vi "Load-lasing-files.vi"(8 "error in (no error)":errorcluster, 11 "Object ref in":T1) -> (0 "error out":errorcluster, 3 "Object ref out":T1)   [LabVIEW 2013, in "SLMControl.lvlib" / "SC-Main.lvclass"]
uses:
  SC-Main.lvclass
  Object-reference.ctl
  SC-Main.lvclass/SC-Main.ctl
  Application-status.ctl
  UI/Control-names.ctl
  Read UI.vi
  Read Status.vi
  Read Base path.vi
  UI/Set-control-boolean.vi
  UI/Set-control-enable-single.vi
  UI/SC-UI.lvclass
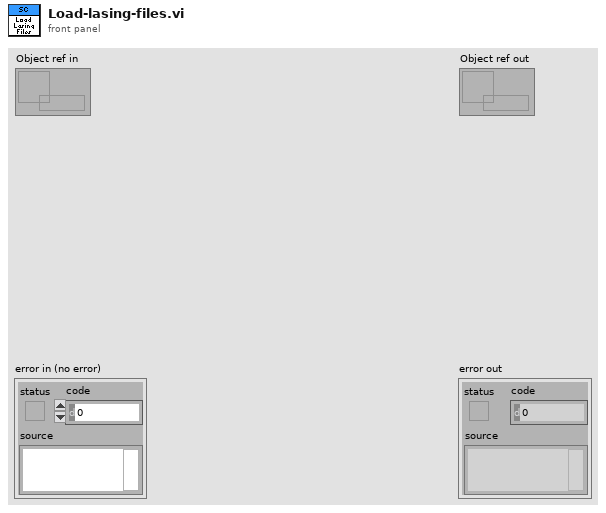
[diagram p1: front panel]
types:
  T1 = typedef "SLMControl.lvlib/SC-Main.lvclass/Object-reference.ctl" = refnum<data-value>
  T2 = typedef "SLMControl.lvlib/SC-UI.lvclass/Control-names.ctl" = enum16{"Com-in", "Com-out", "Help", "Status", "Load configuration", "Save configuration", "Load lasing files", "Load deposition files", "Clear", "Files", "Activate", "Execute", "Abort", "Options", "Current layer", "Current iteration", "Last elapsed time", "Deposition status", "Lasing job", "Status LEDs", "Exiting led", "Initialized led", "Files loaded led", "Activated led", "Executing led", "Deposition led", "Lasing job led", "Lasing led"}
  T3 = typedef "SLMControl.lvlib/SC-Main.lvclass/Application-status.ctl" = enum16{"Idle", "Initialized", "Configured", "Activated", "Started", "Paused", "Stopped", "Reset", "Error", "Exited"}
  T4 = typedef "SLMControl.lvlib/SC-UI.lvclass/Panes-reference.ctl" = refnum<data-value>
  T5 = typedef "SLMControl.lvlib/SC-Main.lvclass/Client-status.ctl" = enum16{"Idle", "Initialized", "Configured", "Activated", "Started", "Paused", "Stopped", "Reset", "Error", "Exited"}
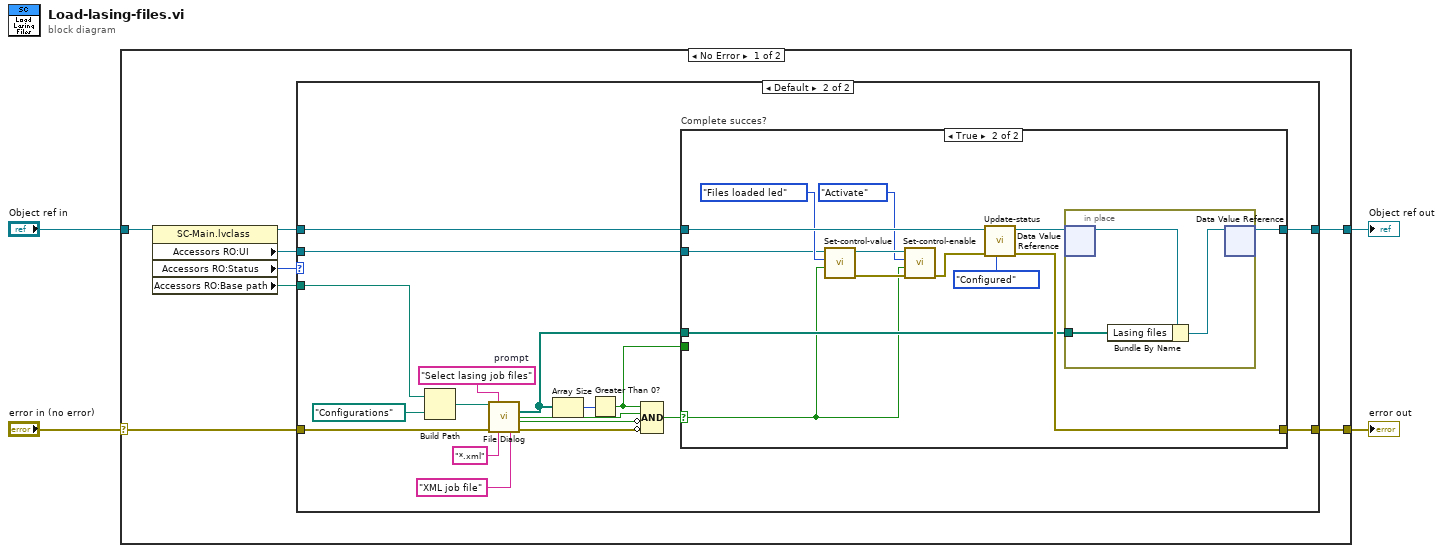
[diagram p0: block diagram]
diagram:
  n1 = case shown="No Error" "error in (no error)" {
    selector: "error in (no error)" -> [w12 w51]
    tunnel: [w8 w51] -> w3
    tunnel: [w7 w50] -> w1
    tunnel: "Object ref in" -> [w11 w50]
    frame No Error {
      n2 = property class="SC-Main.lvclass"(reference=w11) -> (reference out=w9:T1, "Accessors RO:UI"=w10:T4, "Accessors RO:Status"=w6:T5, "Accessors RO:Base path"=w5:path)  [unwired: 1 in, 1 out]
      n3 = case shown="Default" w6 {
        tunnel: w12 -> [w14 w30]
        tunnel: w10 -> [_ w18]
        tunnel: w9 -> [w13 w23]
        tunnel: [w14 w21] -> w8
        tunnel: [w13 w22] -> w7
        tunnel: w5 -> [_ w16]
        frame "Activated".."Paused" {
        }
        frame Default {
          w32 = "Select lasing job files"  # prompt
          n4 = Build Path(base path=w16, name or relative path=path "Configurations") -> (appended path=w17:path)
          n5 = call "File Dialog"("start path"=w17, "prompt"=w32, "error in"=w30, "pattern (all files)"="*.xml", "pattern label"="XML job file") -> ("selected paths"=w20:path[], "exists"=w27:bool, "cancelled"=w26:bool, "error out"=w25:errorcluster)  [unwired: 7 in]
          n6 = Array Size(array=w20) -> (size(s)=w28:i32)
          n7 = Greater Than 0?(x=w28) -> (x > 0?=w19:bool)
          n8 = Compound Arithmetic op=AND(w19, w27, invert w26, invert w25) -> (w24:bool)
          n9 = case "Complete succes?" shown="True" w24 {
            selector: w24 -> [_ w35]
            tunnel: [_ w46] -> w21
            tunnel: [w33 w42] -> w22
            tunnel: w23 -> [w33 w44]
            tunnel: w20 -> [_ w41]
            tunnel: w19 -> [_ _]
            tunnel: w18 -> [_ w36]
            frame False {
            }
            frame True {
              n10 = call-poly "Set-control-value.vi"("Value"=w35, "Control name"=Control-names."Files loaded led", "Panes in"=w36) -> ("error out"=w39:errorcluster, "Panes out"=w38:T4)  [unwired: 7 in]
              n11 = call-poly "Set-control-enable.vi"("error in (no error)"=w39, "Enable?"=w35, "Control name"=Control-names."Activate", "Panes in"=w38) -> ("error out"=w34:errorcluster)  [unwired: 6 in, 1 out]
              n12 = call "Update-status.vi"("Status"=Application-status."Configured", "error in (no error)"=w34, "Object ref in"=w44) -> ("error out"=w46:errorcluster, "Object ref out"=w43:T1)  [unwired: 7 in]
              n13 = in-place {
                in-place-border: w41 -> [w48]
                n14 = in-place-dvr #1(w43) -> (w49:refnum<class "SC-Main.lvclass">)  [unwired: 1 out]
                n15 = Bundle By Name(cluster=w49, "Lasing files"=w48) -> (w47:refnum<class "SC-Main.lvclass">)
                n16 = in-place-dvr #1(w47) -> (w42:T1)  [unwired: 1 out]
              }
            }
          }
        }
      }
    }
    frame Error {
    }
  }
  "error out" <- w3
  "Object ref out" <- w1
